vi "Serialize.vi"(8 "error in":errorcluster, 9 "OwningElement in":refnum<k20>, 10 "Document in":refnum<k20>, 11 "IntergerMeasure in":refnum<class "IntegerMeasure.lvclass">) -> (0 "error out":errorcluster, 1 "OwningElement out":refnum<k20>, 2 "Document out":refnum<k20>, 3 "IntergerMeasure out":refnum<class "IntegerMeasure.lvclass">)   [LabVIEW 2021, in "ProligentXMLGenerator.lvlib" / "IntegerMeasure.lvclass"]
uses:
  IntegerMeasure.lvclass
  IntegerMeasure.lvclass/IntegerMeasure.ctl
  Base/DOMSupport/DOMSupport.lvlib
  Measure/Measure.lvclass
  <vilib>/xml/NI_XML.lvlib
  <vilib>/xml/Close Reference(Node).vi
  MeasureLimit/MeasureLimit.lvclass
  Base/Integer/Integer.lvclass
  Base/Attribute/Attribute.lvclass
  C:/Projects/proligent-xml-generator-labview/src/ProligentXMLGenerator/Measure/Measure/Measure.lvclass
  Base/MeasureKind/MeasureKind.lvclass
  C:/Projects/proligent-xml-generator-labview/src/ProligentXMLGenerator/Base/Attribute/Attribute.lvclass
  C:/Projects/proligent-xml-generator-labview/src/ProligentXMLGenerator/Base/MeasureKind/MeasureKind.lvclass
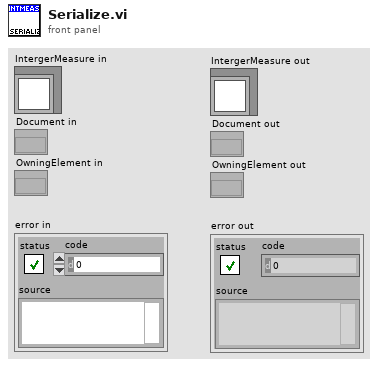
[diagram p1: front panel]
types:
  T1 = typedef "ProligentXMLGenerator.lvlib/IntegerMeasure.lvclass/Data.ctl" = cluster{"Value":refnum<class "Integer.lvclass">}
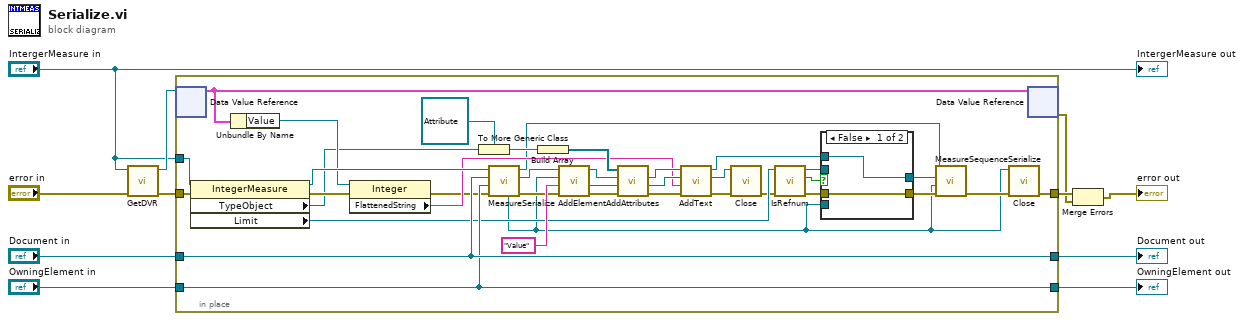
[diagram p0: block diagram]
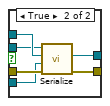
[diagram p2: hidden frame]
diagram:
  n1 = call "GetDVR.vi"("error in"="error in", "IntergerMeasure"="IntergerMeasure in") -> ("error out"=w4:errorcluster, "DVRReference"=w3:refnum<data-value>)  [unwired: 8 in]
  n2 = in-place "In Place Element Structure" {
    in-place-border: [w39] -> w5
    in-place-border: "Document in" -> [w46]
    in-place-border: w4 -> [w45]
    in-place-border: "OwningElement in" -> [w44]
    in-place-border: [w44] -> w7
    in-place-border: [w46] -> w6
    in-place-border: "IntergerMeasure in" -> [w42]
    n3 = in-place-dvr #1(w3) -> (w48:T1)  [unwired: 1 out]
    n4 = property on="Property Node" class="IntegerMeasure"(reference=w42, error in=w45) -> (reference out=w34:refnum<class "IntegerMeasure.lvclass">, error out=w20:errorcluster, "TypeObject"=w16:refnum<class "MeasureKind.lvclass">, "Limit"=w28:refnum<class "MeasureLimit.lvclass">)
    n5 = Unbundle By Name(w48) -> ("Value"=w22:refnum<class "Integer.lvclass">)
    n6 = property on="Property Node" class="Integer"(reference=w22, error in=w20) -> (error out=w19:errorcluster, "FlattenedString"=w21:string)  [unwired: 1 out]
    n7 = To More Generic Class(target class=refnum<class "Attribute.lvclass"> refnum ("ProligentResultProcessor:Attribute"), reference=w16) -> (generic class reference=w17:refnum<class "Attribute.lvclass">)
    n8 = call "MeasureSerialize.vi"("error in"=w19, "OwningElement in"=w44, "Document in"=w46, "Measure in"=w34) -> ("error out"=w32:errorcluster, "Document out"=w33:refnum<k20>, "Measure in"=w14:refnum<class "IntegerMeasure.lvclass">, "Element"=w12:refnum<k20>)  [unwired: 3 in, 1 out]
    n9 = Build Array(w17) -> (w47:refnum<class "Attribute.lvclass">[])
    n10 = call "AddElement.vi"("error in"=w32, "Name"="Value", "OwningElement in"=w12, "Document in"=w33) -> ("error out"=w38:errorcluster, "NewElement"=w40:refnum<k20>, "Document out"=w41:refnum<k20>)  [unwired: 4 in, 1 out]
    n11 = call "AddAttributes.vi"("error in"=w38, "OwningElement in"=w40, "Document in"=w41, "Attributes"=w47) -> ("error out"=w37:errorcluster, "OwningElement out"=w35:refnum<k20>, "Document out"=w36:refnum<k20>)  [unwired: 5 in]
    n12 = call "AddText.vi"("error in"=w37, "Text"=w21, "OwningElement in"=w35, "Document in"=w36) -> ("error out"=w24:errorcluster, "OwningElement out"=w25:refnum<k20>, "Document out"=w27:refnum<k20>)  [unwired: 5 in]
    n13 = call-poly <vilib>:"Close.vi"("error in (no error)"=w24, "node"=w25) -> ("error out"=w23:errorcluster)  [unwired: 7 in]
    n14 = call "IsRefnum.vi"("error in"=w23, "MeasureLimit in"=w28) -> ("error out"=w31:errorcluster, "IsRefnum"=w30:bool, "MeasureLimit out"=w29:refnum<class "MeasureLimit.lvclass">)  [unwired: 7 in]
    n15 = case shown="False" w30 {
      tunnel: w31 -> [w50 w54]
      tunnel: [w50 w56] -> w26
      tunnel: w29 -> [_ w53]
      tunnel: w27 -> [w49 w55]
      tunnel: w12 -> [_ w52]
      tunnel: [w49 w51] -> w13
      frame False {
      }
      frame True {
        n16 = call "Serialize.vi"("error in"=w54, "OwningElement in"=w52, "Document in"=w55, "MeasureLimit in"=w53) -> ("error out"=w56:errorcluster, "Document out"=w51:refnum<k20>)  [unwired: 4 in, 2 out]
      }
    }
    n17 = call "MeasureSequenceSerialize.vi"("error in"=w26, "OwningElement in"=w12, "Document in"=w13, "Measure in"=w14) -> ("error out"=w15:errorcluster)  [unwired: 4 in, 3 out]
    n18 = call-poly <vilib>:"Close.vi"("error in (no error)"=w15, "node"=w12) -> ("error out"=w39:errorcluster)  [unwired: 7 in]
    n19 = in-place-dvr #1(w48) -> (w2:errorcluster)  [unwired: 1 out]
  }
  "Document out" <- w6
  "OwningElement out" <- w7
  n20 = Merge Errors(w5, w2) -> (→"error out":errorcluster)
  "IntergerMeasure out" <- "IntergerMeasure in"
